vi "FPGA Encoder and PWM.vi"() -> ()   [LabVIEW 2019]
uses:
  <vilib>/Platform/TimedLoop/XDataNode/timing_clust.ctl
  <vilib>/Platform/TimedLoop/XDataNode/nitl_modes.ctl
  <vilib>/Platform/TimedLoop/XDataNode/wakeup.ctl
  <vilib>/rvi/Emulation/niFpgaSctlEmulationGetInTimedLoop.vi
  <vilib>/rvi/Emulation/niFpgaEmulationReportErrorSimple.vi
  <vilib>/rvi/Emulation/niFpgaGetClockAttributes.vi
  <vilib>/rvi/Emulation/niFpgaCriticalErrorInLSC.vi
  <vilib>/rvi/eio/common/nirviEmuTemplateMethod_errors.vi
  <vilib>/rvi/Emulation/niFpgaProcessEmulError.vi
  <vilib>/Platform/TimedLoop/XDataNode/XDataNode.xnode
  <vilib>/eio/EIONode/EIONode.xnode
  <vilib>/Platform/TimedLoop/XDataNode/XDNodeRunTimeDep.lvlib
panel:
  out "Motor 2 Encoder Position":i32=4864
  out "Motor 2 Encoder Period":i32=2147483647
  in  "Reset Encoder Position":bool
  out "Motor 1 Encoder Position":i32=-45520
  out "Motor 1 Encoder Period":i32=2147483647
  in  "Motor 2 Duty Cycle":i16
  in  "Motor 1 Duty Cycle":i16
  in  "Motor Duty Cycle Period":i16=2000
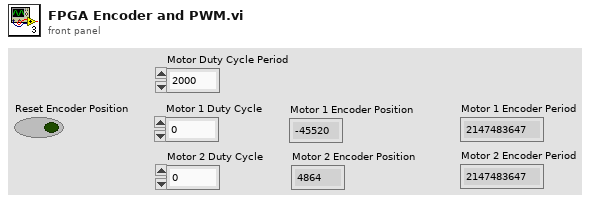
[diagram p1: front panel]
types:
  T1 = typedef "XDNodeRunTimeDep.lvlib/timing_clust.ctl" = cluster{"Expected End [f-1]":u64, "Actual End [f-1]":u64, "Finished Late? [f-1]":bool, "Expected End [i-1]":u64, "Actual End [i-1]":u64, "Finished Late? [i-1]":bool, "Expected Start [i]":u64, "Actual Start [i]":u64, "Expected Start [f]":u64, "Actual Start [f]":u64, "Source Name":string, "Structure Name":string, "Period":i64, "Deadline":i64, "Offset":i64, "Start":i64, "Priority":i32, "Timeout":i32, "Mode":T2, "Wakeup Reason":T3, "Error":errorcluster, "Source Type":string, "Secondary Source Type":string, "Global End Time":u64, "Global Start Time":u64, "Frame Duration":u64, "Iteration Duration":u64, "Assigned CPU":i32, "I/O Scan Engine Mode":u32}
  T2 = typedef "XDNodeRunTimeDep.lvlib/nitl_modes.ctl" = enum32{"No Change", "Process missed periods, maintain original phase", "Discard missed periods, maintain original phase", "Process missed periods, ignore original phase", "Discard missed periods, ignore original phase"}
  T3 = typedef "XDNodeRunTimeDep.lvlib/wakeup.ctl" = enum32{"Normal", "Aborted", "Asynchronous wakeup", "Timing source error", "Timed loop error", "Timeout"}
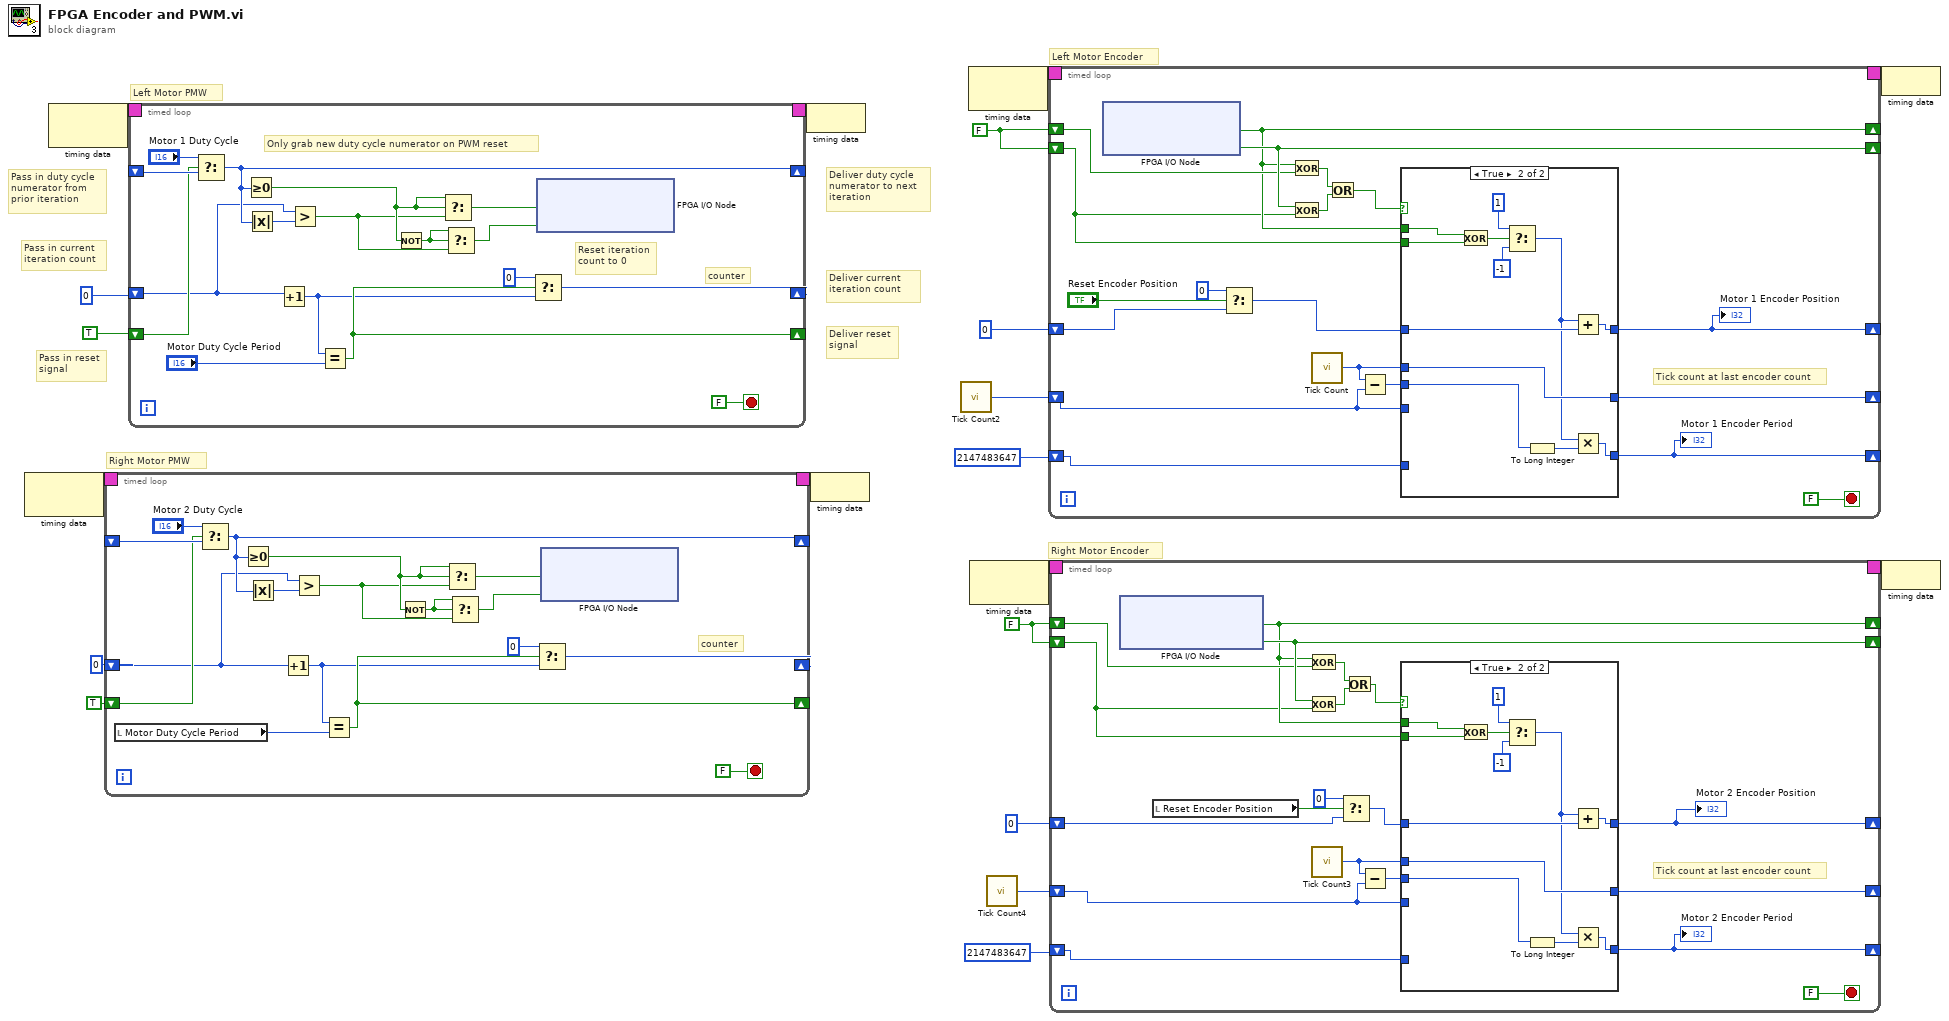
[diagram p0: block diagram]
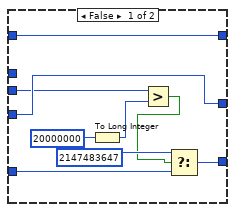
[diagram p2: hidden frame]
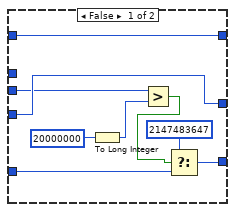
[diagram p3: hidden frame]
diagram:
  w4 = FALSE
  w10 = FALSE
  # "Deliver reset signal"
  # "Pass in reset signal"
  # "Deliver current iteration count"
  # "Pass in current iteration count"
  # "Deliver duty cycle numerator to next iteration"
  # "Pass in duty cycle numerator from prior iteration"
  # "Right Motor PMW"
  # "Right Motor Encoder"
  # "Left Motor Encoder"
  # "Left Motor PMW"
  n1 = node-c288() -> (w18:T1)  [unwired: 1 in]
  n2 = node-c288() -> (w20:T1)  [unwired: 1 in]
  n3 = timed-loop {
    timing: w18 -> [_]
    timing-out: [_] -> w17
    shift-right: [w34] -> _
    shift-left: _ -> [w36]
    shift-right: [w31] -> _
    shift-left: TRUE -> [w35]
    shift-right: [w33] -> _
    shift-left: i16 0 -> [w23]
    stop <- FALSE stop-if-true
    # "counter"
    n4 = local read "Motor Duty Cycle Period"() -> (w21:i16)
    n5 = Select(t="Motor 2 Duty Cycle", s=w35, f=w36) -> (s? t:f=w34:i16)
    n6 = Greater Or Equal To 0?(x=w34) -> (x >= 0?=w26:bool)
    n7 = Absolute Value(x=w34) -> (abs(x)=w24:i16)
    n8 = Increment(x=w23) -> (x+1=w30:i16)
    n9 = Greater?(x=w23, y=w24) -> (0:w22:bool)
    n10 = Equal?(x=w30, y=w21) -> (x = y?=w31:bool)
    n11 = Not(x=w26) -> (.not. x?=w25:bool)
    n12 = Select(t=w26, s=w26, f=w22) -> (s? t:f=w28:bool)
    n13 = Select(t=w25, s=w25, f=w22) -> (s? t:f=w27:bool)
    n14 = Select(t=i16 0, s=w31, f=w30) -> (s? t:f=w33:i16)
    n15 = xnode "FPGA I/O Node"("ConnectorB/DIO2"=w28, "ConnectorB/DIO3"=w27) -> ()  [unwired: 2 in, 2 out]
  }
  n16 = timed-loop {
    timing: w20 -> [_]
    timing-out: [_] -> w19
    shift-right: [w53] -> _
    shift-left: _ -> [w55]
    shift-right: [w50] -> _
    shift-left: TRUE -> [w54]
    shift-right: [w52] -> _
    shift-left: i16 0 -> [w42]
    stop <- FALSE stop-if-true
    # "Reset iteration count to 0"
    # "Only grab new duty cycle numerator on PWM reset"
    # "counter"
    n17 = Select(t="Motor 1 Duty Cycle", s=w54, f=w55) -> (s? t:f=w53:i16)
    n18 = Greater Or Equal To 0?(x=w53) -> (x >= 0?=w45:bool)
    n19 = Absolute Value(x=w53) -> (abs(x)=w43:i16)
    n20 = Increment(x=w42) -> (x+1=w49:i16)
    n21 = Greater?(x=w42, y=w43) -> (0:w41:bool)
    n22 = Equal?(x=w49, y="Motor Duty Cycle Period") -> (x = y?=w50:bool)
    n23 = Not(x=w45) -> (.not. x?=w44:bool)
    n24 = Select(t=w45, s=w45, f=w41) -> (s? t:f=w47:bool)
    n25 = Select(t=w44, s=w44, f=w41) -> (s? t:f=w46:bool)
    n26 = Select(t=i16 0, s=w50, f=w49) -> (s? t:f=w52:i16)
    n27 = xnode ("FPGA I/O Node")("ConnectorB/DIO0"=w47, "ConnectorB/DIO1"=w46) -> ()  [unwired: 2 in, 2 out]
  }
  n28 = node-c288(w19) -> ()
  n29 = node-c288(w17) -> ()
  n30 = call "Tick Count2"() -> ("Tick Count(Ticks)"=w8:u32)
  n31 = node-c288() -> (w12:T1)  [unwired: 1 in]
  n32 = node-c288() -> (w6:T1)  [unwired: 1 in]
  n33 = call "Tick Count4"() -> ("Tick Count(Ticks)"=w2:u32)
  n34 = timed-loop {
    timing: w12 -> [_]
    timing-out: [_] -> w11
    shift-right: [w72] -> _
    shift-left: w10 -> [w73]
    shift-right: [w74] -> _
    shift-left: w10 -> [w71]
    shift-right: [w67] -> _
    shift-left: 0 -> [w69]
    shift-right: [w66] -> _
    shift-left: w8 -> [w63]
    shift-right: [w61] -> _
    shift-left: 2147483647 -> [w62]
    stop <- FALSE stop-if-true
    # "Tick count at last encoder count"
    n35 = xnode "FPGA I/O Node"() -> ("ConnectorB/DIO6"=w72:bool, "ConnectorB/DIO7"=w74:bool)  [unwired: 2 in, 2 out]
    n36 = Select(t=0, s="Reset Encoder Position", f=w69) -> (s? t:f=w68:i32)
    n37 = Exclusive Or(1:w73, 2:w72) -> (0:w76:bool)
    n38 = Exclusive Or(1:w71, 2:w74) -> (0:w75:bool)
    n39 = call "Tick Count"() -> ("Tick Count(Ticks)"=w65:u32)
    n40 = Or(x=w76, y=w75) -> (x .or. y?=w77:bool)
    n41 = Subtract(x=w65, y=w63) -> (x-y=w64:u32)
    n42 = case shown="True" w77 {
      tunnel: w72 -> [_ w98]
      tunnel: w71 -> [_ w97]
      tunnel: w68 -> [w86 w94]
      tunnel: [w86 w95] -> w67
      tunnel: w65 -> [_ w91]
      tunnel: [w85 w91] -> w66
      tunnel: w64 -> [w84 w88]
      tunnel: w63 -> [w85 _]
      tunnel: w62 -> [w79 _]
      tunnel: [w78 w87] -> w61
      frame False {
        n43 = To Long Integer(number=20000000) -> (32bit integer=w82:i32)
        n44 = Greater?(x=w84, y=w82) -> (0:w80:bool)
        n45 = Select(t=2147483647, s=w80, f=w79) -> (s? t:f=w78:i32)
      }
      frame True {
        n46 = Exclusive Or(1:w97, 2:w98) -> (0:w96:bool)
        n47 = Select(t=1, s=w96, f=-1) -> (s? t:f=w90:i32)
        n48 = To Long Integer(number=w88) -> (32bit integer=w89:i32)
        n49 = Add(x=w90, y=w94) -> (x+y=w95:i32)
        n50 = Multiply(x=w90, y=w89) -> (x*y=w87:i32)
      }
    }
    "Motor 1 Encoder Position" <- w67
    "Motor 1 Encoder Period" <- w61
  }
  n51 = timed-loop {
    timing: w6 -> [_]
    timing-out: [_] -> w5
    shift-right: [w114] -> _
    shift-left: w4 -> [w115]
    shift-right: [w116] -> _
    shift-left: w4 -> [w113]
    shift-right: [w109] -> _
    shift-left: 0 -> [w111]
    shift-right: [w108] -> _
    shift-left: w2 -> [w105]
    shift-right: [w103] -> _
    shift-left: 2147483647 -> [w104]
    stop <- FALSE stop-if-true
    # "Tick count at last encoder count"
    n52 = xnode "FPGA I/O Node"() -> ("ConnectorB/DIO11"=w114:bool, "ConnectorB/DIO12"=w116:bool)  [unwired: 2 in, 2 out]
    n53 = local read "Reset Encoder Position"() -> (w101:bool)
    n54 = Exclusive Or(1:w115, 2:w114) -> (0:w118:bool)
    n55 = Exclusive Or(1:w113, 2:w116) -> (0:w117:bool)
    n56 = call "Tick Count3"() -> ("Tick Count(Ticks)"=w107:u32)
    n57 = Select(t=0, s=w101, f=w111) -> (s? t:f=w110:i32)
    n58 = Or(x=w118, y=w117) -> (x .or. y?=w119:bool)
    n59 = Subtract(x=w107, y=w105) -> (x-y=w106:u32)
    n60 = case shown="True" w119 {
      tunnel: w114 -> [_ w140]
      tunnel: w113 -> [_ w139]
      tunnel: w110 -> [w128 w136]
      tunnel: [w128 w137] -> w109
      tunnel: w107 -> [_ w133]
      tunnel: [w127 w133] -> w108
      tunnel: w106 -> [w126 w130]
      tunnel: w105 -> [w127 _]
      tunnel: w104 -> [w121 _]
      tunnel: [w120 w129] -> w103
      frame False {
        n61 = To Long Integer(number=20000000) -> (32bit integer=w124:i32)
        n62 = Greater?(x=w126, y=w124) -> (0:w122:bool)
        n63 = Select(t=2147483647, s=w122, f=w121) -> (s? t:f=w120:i32)
      }
      frame True {
        n64 = Exclusive Or(1:w139, 2:w140) -> (0:w138:bool)
        n65 = Select(t=1, s=w138, f=-1) -> (s? t:f=w132:i32)
        n66 = To Long Integer(number=w130) -> (32bit integer=w131:i32)
        n67 = Add(x=w132, y=w136) -> (x+y=w137:i32)
        n68 = Multiply(x=w132, y=w131) -> (x*y=w129:i32)
      }
    }
    "Motor 2 Encoder Position" <- w109
    "Motor 2 Encoder Period" <- w103
  }
  n69 = node-c288(w11) -> ()
  n70 = node-c288(w5) -> ()
